vi "GetEventRegRefnum.vi"(8 "error in":errorcluster, 11 "message ref in":refnum<class "CLM_LocalMessage_UserEvent.lvclass">) -> (0 "error out":errorcluster, 2 "reg refnum":refnum<event-registration>, 3 "message ref out":refnum<class "CLM_LocalMessage_UserEvent.lvclass">)   [LabVIEW 2013, in "CLM_LocalMessage_UserEvent.lvclass"]
uses:
  CLM_LocalMessage_UserEvent.lvclass
  MessageUserEvent.ctl
  LocalMessage/Message.ctl
  CLM_LocalMessage_UserEvent.lvclass/CLM_LocalMessage_UserEvent.ctl
  LocalMessage/CLM_LocalMessage.lvclass
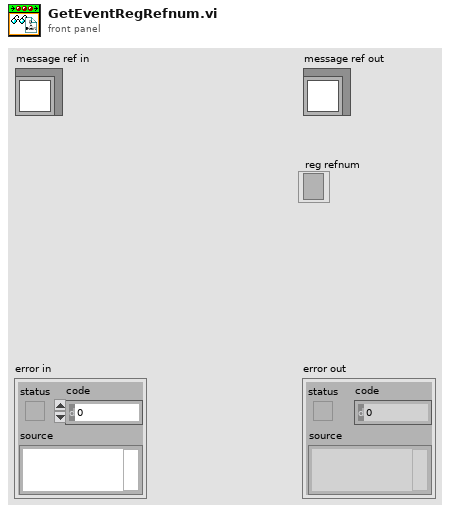
[diagram p1: front panel]
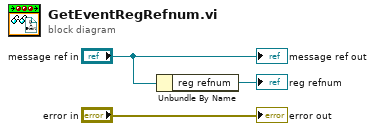
[diagram p0: block diagram]
diagram:
  n1 = Unbundle By Name("message ref in") -> ("reg refnum"=→"reg refnum":refnum<event-registration>)
  "error out" <- "error in"
  "message ref out" <- "message ref in"
